vi "LSX Set Process Messages Proc.vi"(8 "error in (no error)":errorcluster, 10 "pProc":u32, 11 "lLSID":i32) -> (0 "error out":errorcluster, 2 "pProc out":u32, 3 "function return":i32)   [LabVIEW 2018, in "Tango.lvlib"]
doc: "TANGOAPI int TANGOCALL LSX_SetProcessMessagesProc (int lLSID, void* pProc);"
uses:
  Tango.lvlib
  SubVIs/Tango_DLL.dll
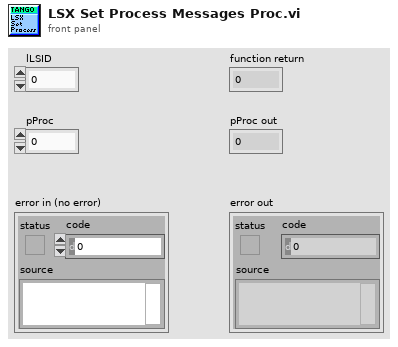
[diagram p1: front panel]
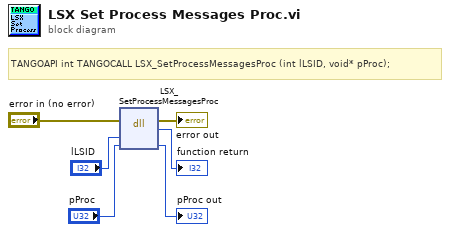
[diagram p0: block diagram]
diagram:
  # "TANGOAPI int TANGOCALL LSX_SetProcessMessagesProc (int lLSID, void* pProc);"
  n1 = dll-call lib="C:/Users/Familie/Documents/LabviewIX81/lib/TANGO Stage/SubVIs/Tango_DLL.*" fn="LSX_SetProcessMessagesProc"(error in="error in (no error)", "lLSID"="lLSID", "pProc"="pProc") -> (error out=→"error out":errorcluster, →"function return":i32, "pProc"=→"pProc out":u32)  [unwired: 3 in, 1 out]
